vi "Write Log Warnings_.vi"(8 "error in (no error)":errorcluster, 10 "Log Warnings?":bool, 11 "System Log in":refnum<class "System Log.lvclass">) -> (0 "error out":errorcluster, 3 "System Log out":refnum<class "System Log.lvclass">)   [LabVIEW 2016, in "System Log.lvclass"]
uses:
  System Log.lvclass
  System Log.lvclass/System Log.ctl
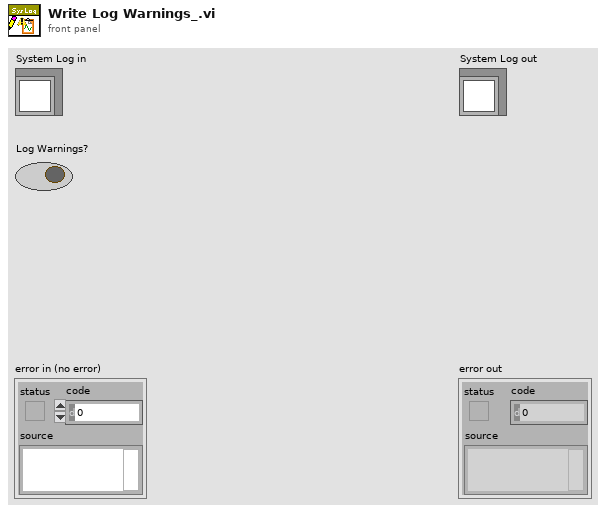
[diagram p1: front panel]
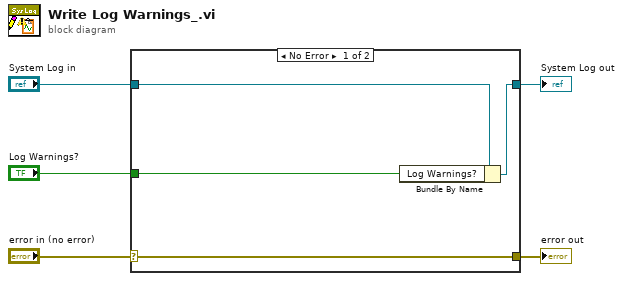
[diagram p0: block diagram]
diagram:
  n1 = case shown="No Error" "error in (no error)" {
    selector: "error in (no error)" -> [w9 w10]
    tunnel: [w9 w10] -> w4
    tunnel: [w7 w11] -> w2
    tunnel: "System Log in" -> [w8 w11]
    tunnel: "Log Warnings?" -> [w6 _]
    frame No Error {
      n2 = Bundle By Name(cluster=w8, "Log Warnings?"=w6) -> (w7:refnum<class "System Log.lvclass">)
    }
    frame Error {
    }
  }
  "error out" <- w4
  "System Log out" <- w2
